vi "dvp Vi Get Ae Mode.vi"(10 "pAeMode":u32(ring) items=["AE_MODE_AE_AG", "AE_MODE_AG_AE", "AE_MODE_AE_ONLY", "AE_MODE_AG_ONLY"], 11 "handle":u32) -> (2 "pAeMode out":u32(ring) items=["AE_MODE_AE_AG", "AE_MODE_AG_AE", "AE_MODE_AE_ONLY", "AE_MODE_AG_ONLY"], 3 "function return":u32(ring))   [LabVIEW 2018, in "LabViewDVPCamera.lvlib"]
doc: "LabviewDvp2Api dvpStatus dvpViGetAeMode(dvpHandle handle, dvpAeMode *pAeMode);"
uses:
  LabViewDVPCamera.lvlib
  LabViewDVPCamera/LabViewDVPCamera.dll
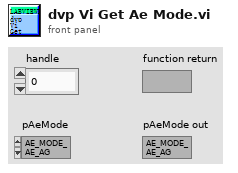
[diagram p1: front panel]
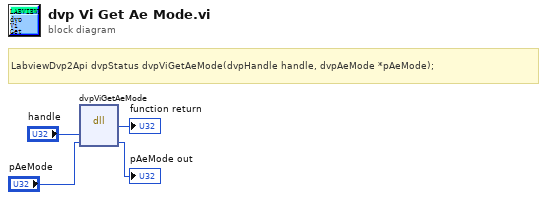
[diagram p0: block diagram]
diagram:
  # "LabviewDvp2Api dvpStatus dvpViGetAeMode(dvpHandle handle, dvpAeMode *pAeMode);"
  n1 = dll-call lib="C:/Program Files (x86)/DVP2 Labview cn 64/Sample/LabViewDVPCamera/LabViewDVPCamera.*" fn="dvpViGetAeMode"("handle"="handle", "pAeMode"="pAeMode") -> (→"function return":u32, "pAeMode"=→"pAeMode out":u32)  [unwired: 4 in, 2 out]
